vi "Fit Result to String.vi"(8 "error in (no error)":errorcluster, 11 "Exponential Fit in":refnum<class "Exponential Fit.lvclass">) -> (0 "error out":errorcluster, 2 "Array":string[](array[string]), 3 "Exponential Fit out":refnum<class "Exponential Fit.lvclass">)   [LabVIEW 2016, in "Exponential Fit.lvclass"]
uses:
  Exponential Fit.lvclass
  Exponential Fit.lvclass/Exponential Fit.ctl
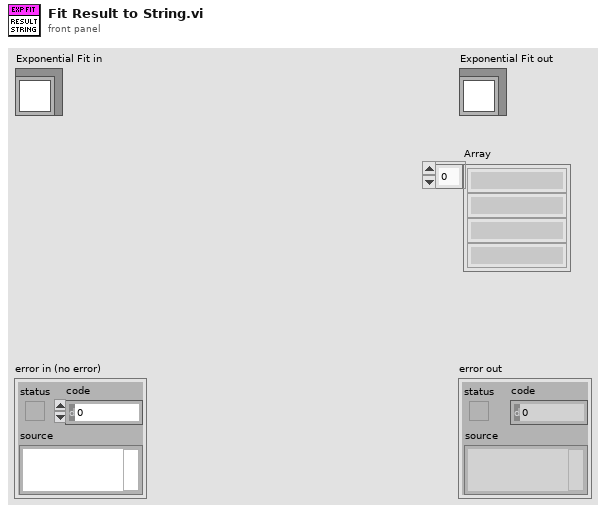
[diagram p1: front panel]
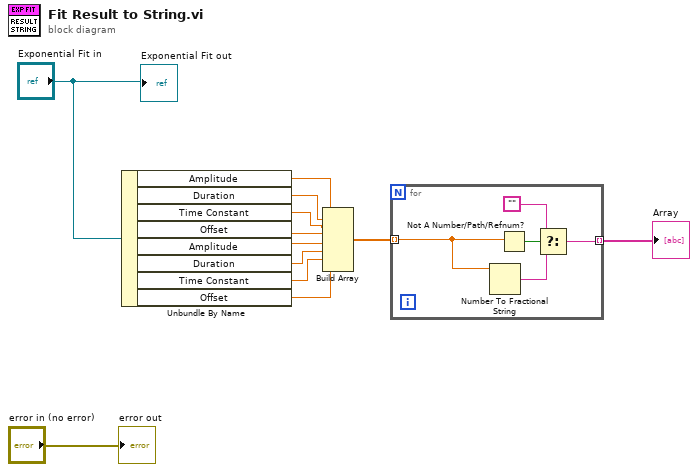
[diagram p0: block diagram]
diagram:
  n1 = Unbundle By Name("Exponential Fit in") -> ("Amplitude"=w10:dbl, "Duration"=w9:dbl, "Time Constant"=w8:dbl, "Offset"=w7:dbl, "Amplitude"=w6:dbl, "Duration"=w5:dbl, "Time Constant"=w4:dbl, "Offset"=w3:dbl)
  n2 = Build Array(w10, w9, w8, w7, w6, w5, w4, w3) -> (w2:dbl[])
  n3 = for {
    tunnel: [w17] -> w1 mode=indexing
    tunnel: w2 -> [w13] mode=indexing
    n4 = Number To Fractional String(number=w13) -> (F-format string=w14:string)  [unwired: 3 in]
    n5 = Not A Number/Path/Refnum?(number/path/refnum=w13) -> (NaN/Path/Refnum?=w16:bool)
    n6 = Select(t="", s=w16, f=w14) -> (s? t:f=w17:string)
  }
  "Array" <- w1
  "error out" <- "error in (no error)"
  "Exponential Fit out" <- "Exponential Fit in"
